vi "Multi bin files-Obtain frame number and location.vi"(8 "error in (no error)":errorcluster, 10 "Funct data structure":bool, 11 "Cam Binary Videos paths":path[](array[path])=[path "F:/UCL/Rig 3 MovCor integration version/Datasets/150623_21_01_30 TimeLapse-Test set-sw trig/150623_21_01_30 TimeLapse VidRec/BodyCam.bin", path "F:/UCL/Rig 3 MovCor integration version/Datasets/150623_21_01_30 TimeLapse-Test set-sw trig/150623_21_01_30 TimeLapse VidRec/EyeCam.bin", path "F:/UCL/Rig 3 MovCor integration version/Datasets/150623_21_01_30 TimeLapse-Test set-sw trig/150623_21_01_30 TimeLapse VidRec/WhiskersCam.bin"]) -> (0 "Error out":errorcluster, 3 "Frame numbers & locations in each video file":T1[](array[typedef]))   [LabVIEW 2020]
uses:
  Typedefs/Number of frames and locations cluster.ctl
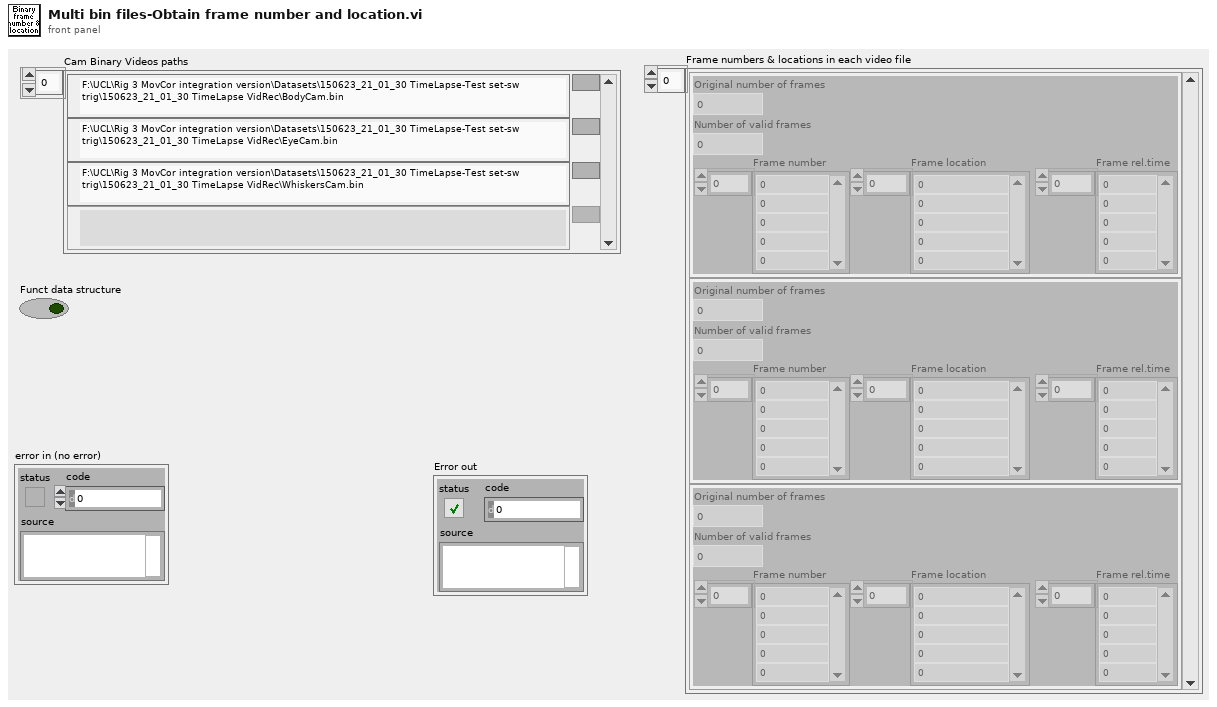
[diagram p1: front panel]
types:
  T1 = typedef "Number of frames and locations cluster.ctl" = cluster{"Original number of frames":i32, "Number of valid frames":i32, "Frame number":i64[], "Frame location":i64[], "Frame rel.time":i64[]}
  T2 = typedef "Test header stats cluster.ctl" = cluster{"Number of acquired data-points":dbl, "Acquisition time (ms)":dbl, "Number of acquired frames":dbl}
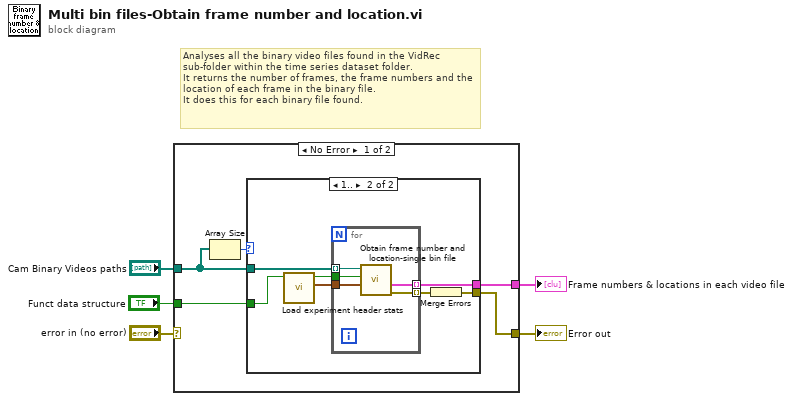
[diagram p0: block diagram]
diagram:
  # "Analyses all the binary video files found in the VidRec sub-folder within the time series dataset folder.\nIt returns the number of frames, the frame numbers and the location of each frame in the binary file.\nIt does this for each binary file found."
  n1 = case shown="No Error" "error in (no error)" {
    selector: "error in (no error)" -> [_ w23]
    tunnel: [w10 _] -> w1
    tunnel: [w9 w23] -> w5
    tunnel: "Cam Binary Videos paths" -> [w8 _]
    tunnel: "Funct data structure" -> [w6 _]
    frame No Error {
      n2 = Array Size(array=w8) -> (size(s)=w7:i32)
      n3 = case shown="1.." w7 {
        tunnel: w8 -> [_ w14]
        tunnel: [_ w17] -> w10
        tunnel: [_ w15] -> w9
        tunnel: w6 -> [_ w11]
        frame Default {
        }
        frame 1.. {
          n4 = call "Load experiment header stats.vi"("Funct data structure"=w11) -> ("Experiment Header's Statistics"=w13:T2, "Acquisition time unknown"=w12:bool)  [unwired: 9 in]
          n5 = for {
            tunnel: w14 -> [w22] mode=indexing
            tunnel: [w21] -> w17 mode=indexing
            tunnel: [w20] -> w16 mode=indexing
            tunnel: w13 -> [w19]
            tunnel: w12 -> [w18]
            n6 = call "Obtain frame number and location-single bin file.vi"("Experiment Header's Statistics"=w19, "Acquisition time unknown"=w18, "Binary file to read"=w22) -> ("error out"=w20:errorcluster, "Frame numbers & locations"=w21:T1)  [unwired: 7 in]
          }
          n7 = Merge Errors(w16) -> (w15:errorcluster)
        }
      }
    }
    frame Error {
    }
  }
  "Error out" <- w5
  "Frame numbers & locations in each video file" <- w1
